vi "CSDB_Config.write SV CSV-file.vi"(1 "objects":cluster{"INSTANCENAME":string, "Class":string}[](array[cluster])=[{"INSTANCENAME"="FOPICAEN1.Board00.Chan000", "Class"=""}], 5 "error in":errorcluster) -> (19 "error out":errorcluster)   [LabVIEW 2014, in "CSDB_Config.lvlib"]
doc: "Writes a CSV file of Shared Variable definitions that can be used for importing into DSCIntProc class."
uses:
  CSDB_Config.lvlib
  Instance           1 37Saved   CSDB_Config.write SV CSV-file .vi
  CSlibraries/UtilityLib/UtilityLib.lvlib
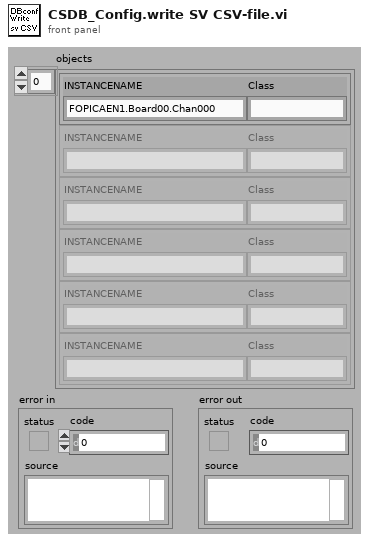
[diagram p1: front panel]
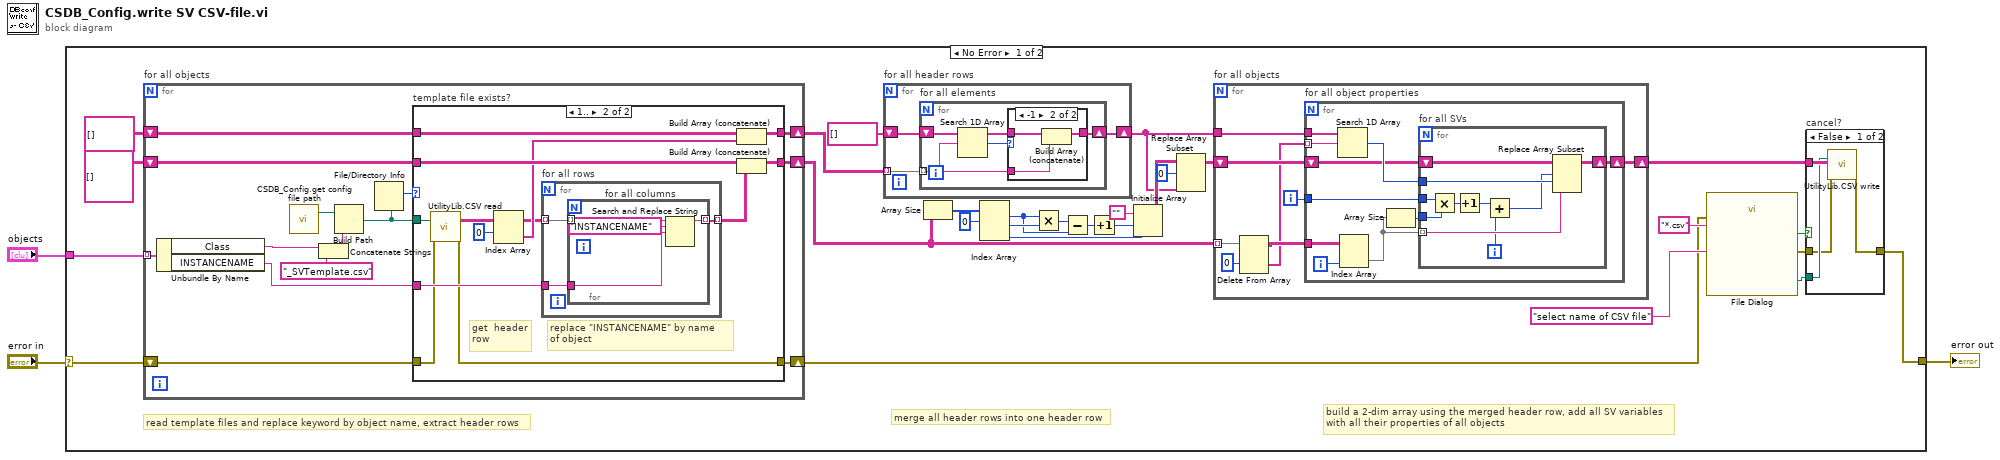
[diagram p0: block diagram]
diagram:
  n1 = case shown="No Error" "error in" {
    selector: "error in" -> [w24 w112]
    tunnel: "objects" -> [w31 _]
    tunnel: [w25 w112] -> w2
    frame No Error {
      # "build a 2-dim array using the merged header row, add all SV variables\nwith all their properties of all objects"
      # "merge all header rows into one header row"
      # "read template files and replace keyword by object name, extract header rows"
      n2 = for "for all objects" {
        tunnel: w31 -> [w89] mode=indexing
        shift-right: [w82] -> w17
        shift-left: string[][][] [] -> [w81]
        shift-right: [w78] -> w28
        shift-left: string[][] [] -> [w79]
        shift-right: [w77] -> w20
        shift-left: w24 -> [w76]
        n3 = Unbundle By Name(w89) -> ("Class"=w88:string, "INSTANCENAME"=w80:string)
        n4 = call "CSDB_Config.get config file path.vi"() -> ("config file path"=w84:path)  [unwired: 18 in, 1 out]
        n5 = Concatenate Strings(w88, "_SVTemplate.csv" ("string")) -> (w86:string)
        n6 = Build Path(base path=w84, name or relative path=w86) -> (appended path=w85:path)
        n7 = File/Directory Info(path=w85) -> (size=w83:i64)  [unwired: 1 in, 6 out]
        n8 = case "template file exists?" shown="1.." w83 {
          tunnel: w85 -> [_ w104]
          tunnel: [w92 w103] -> w82
          tunnel: w81 -> [w92 w102]
          tunnel: w80 -> [_ w101]
          tunnel: w79 -> [w91 w99]
          tunnel: [w91 w98] -> w78
          tunnel: w76 -> [w90 w95]
          tunnel: [w90 w94] -> w77
          frame 0, Default {
          }
          frame 1.. {
            # "replace \"INSTANCENAME\" by name\nof object"
            # "get  header\nrow"
            n9 = call "UtilityLib.CSV read.vi"("file (use dialog)"=w104, "error in"=w95) -> ("CSVArray"=w96:string[][], "error out"=w94:errorcluster)  [unwired: 16 in]
            n10 = Index Array(array=w96, index (row)=0) -> (element=w97:string[])  [unwired: 1 in]
            n11 = for "for all rows" {
              tunnel: w96 -> [w107] mode=indexing
              tunnel: w101 -> [w106]
              tunnel: [w105] -> w100 mode=indexing
              n12 = for "for all columns" {
                tunnel: w107 -> [w111] mode=indexing
                tunnel: w106 -> [w109]
                tunnel: [w108] -> w105 mode=indexing
                n13 = Search and Replace String(input string=w111, search string="INSTANCENAME", replace string=w109) -> (result string=w108:string)  [unwired: 5 in, 3 out]
              }
            }
            n14 = Build Array (concatenate)(w99, w97) -> (w98:string[][])
            n15 = Build Array (concatenate)(w102, w100) -> (w103:string[][][])
          }
        }
      }
      n16 = for "for all header rows" {
        tunnel: w28 -> [w67] mode=indexing
        shift-right: [w65] -> w6
        shift-left: string[] [] -> [w66]
        n17 = for "for all elements" {
          tunnel: w67 -> [w68] mode=indexing
          shift-right: [w69] -> w65
          shift-left: w66 -> [w70]
          n18 = Search 1D Array(1D array=w70, element=w68) -> (index of element=w71:i32)  [unwired: 1 in]
          n19 = case shown="-1" w71 {
            tunnel: w70 -> [w72 w75]
            tunnel: [w72 w73] -> w69
            tunnel: w68 -> [_ w74]
            frame 0, Default {
            }
            frame -1 {
              n20 = Build Array (concatenate)(w75, w74) -> (w73:string[])
            }
          }
        }
      }
      n21 = Array Size(array=w17) -> (size(s)=w15:i32[])
      n22 = Index Array(array=w15, index #1=0 ("index")) -> (element #1=w11:i32, element #2=w13:i32, element #3=w8:i32)  [unwired: 2 in]
      n23 = Multiply(x=w11, y=w13) -> (x*y=w12:i32)
      n24 = Subtract(x=w12, y=w11) -> (x-y=w10:i32)
      n25 = Increment(x=w10) -> (x+1=w9:i32)
      n26 = Initialize Array("", w9, w8) -> (w7:string[][])
      n27 = Replace Array Subset(array=w7, new element=w6, index (row)=0) -> (w4:string[][])  [unwired: 1 in]
      n28 = for "for all objects" {
        tunnel: w17 -> [w40] mode=indexing
        shift-right: [w42] -> w26
        shift-left: w4 -> [w43]
        tunnel: w6 -> [w44]
        i -> [w41]
        n29 = Delete From Array(array=w40, index (row)=0) -> (deleted portion=w37:string[], array with subset deleted=w39:string[][])  [unwired: 2 in]
        n30 = for "for all object properties" {
          tunnel: w37 -> [w53] mode=indexing
          tunnel: w44 -> [w54]
          tunnel: w39 -> [w52]
          shift-right: [w51] -> w42
          shift-left: w43 -> [w49]
          tunnel: w41 -> [w47]
          i -> [w48]
          n31 = Search 1D Array(1D array=w54, element=w53) -> (index of element=w50:i32)  [unwired: 1 in]
          n32 = Index Array(array=w52, index (col)=w48) -> (element=w46:string[])  [unwired: 1 in]
          n33 = Array Size(array=w46) -> (size(s)=w45:i32)
          n34 = for "for all SVs" {
            tunnel: w50 -> [w61]
            shift-right: [w63] -> w51
            shift-left: w49 -> [w64]
            tunnel: w46 -> [w62] mode=indexing
            tunnel: w47 -> [w58]
            tunnel: w45 -> [w57]
            i -> [w60]
            n35 = Multiply(x=w58, y=w57) -> (x*y=w56:i32)
            n36 = Increment(x=w56) -> (x+1=w55:i32)
            n37 = Add(x=w55, y=w60) -> (x+y=w59:i32)
            n38 = Replace Array Subset(array=w64, new element=w62, index (row)=w59, index (col)=w61) -> (w63:string[][])
          }
        }
      }
      n39 = call "File Dialog"("prompt"="select name of CSV file", "error in"=w20, "pattern (all files)"="*.csv") -> ("selected path"=w23:path, "cancelled"=w18:bool, "error out"=w19:errorcluster)  [unwired: 9 in, 1 out]
      n40 = case "cancel?" shown="False" w18 {
        tunnel: w26 -> [w35 _]
        tunnel: [w34 w36] -> w25
        tunnel: w23 -> [w33 _]
        tunnel: w19 -> [w32 w36]
        frame False {
          n41 = call "UtilityLib.CSV write.vi"("file (use dialog)"=w33, "CSVArray"=w35, "error in"=w32) -> ("error out"=w34:errorcluster)  [unwired: 16 in]
        }
        frame True {
        }
      }
    }
    frame Error {
    }
  }
  "error out" <- w2
